vi "Update exp names list.vi"(8 "error in (no error)":errorcluster, 9 "# row":i32, 10 "Experiment in":refnum<class "Experiment.lvclass">, 11 "Control-Client in":refnum<class "Control-Client.lvclass">) -> (0 "error out":errorcluster, 3 "Control-Client out":refnum<class "Control-Client.lvclass">)   [LabVIEW 2019, in "Control-Client.lvclass"]
uses:
  Control-Client.lvclass
  Experiments/Experiment.lvclass
  Control-Client.lvclass/Control-Client.ctl
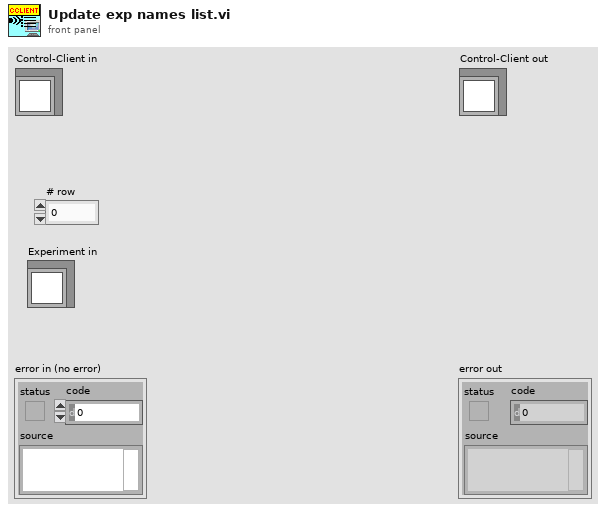
[diagram p1: front panel]
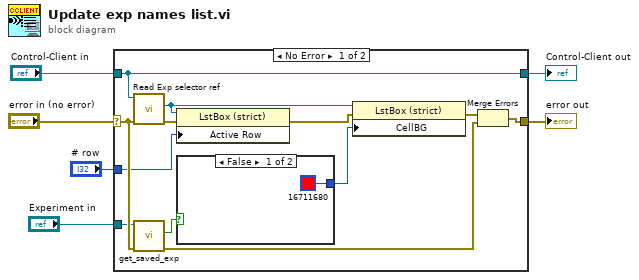
[diagram p0: block diagram]
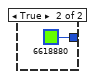
[diagram p2: hidden frame]
diagram:
  n1 = case shown="No Error" "error in (no error)" {
    selector: "error in (no error)" -> [w16 w22]
    tunnel: [w11 w22] -> w5
    tunnel: [w15 w21] -> w3
    tunnel: "Control-Client in" -> [w15 w21]
    tunnel: "Experiment in" -> [w8 _]
    tunnel: "# row" -> [w7 _]
    frame No Error {
      n2 = call "Read Exp selector ref.vi"("error in (no error)"=w16, "Control-Client in"=w15) -> ("error out"=w14:errorcluster, "Exp selector ref"=w18:refnum<vi>)  [unwired: 7 in, 1 out]
      n3 = call "get_saved_exp.vi"("error in (no error)"=w16, "Experiment.lvclass in"=w8) -> ("error out"=w10:errorcluster, "Saved"=w17:bool)  [unwired: 7 in, 1 out]
      n4 = property on="Property Node" class="LstBox (strict)"(reference=w18, error in=w14, "Active Row"=w7) -> (error out=w13:errorcluster)  [unwired: 1 out]
      n5 = case shown="False" w17 {
        tunnel: [u32 16711680 u32 6618880] -> w9
        frame False {
        }
        frame True {
        }
      }
      n6 = property on="Property Node" class="LstBox (strict)"(reference=w18, error in=w13, "CellBG"=w9) -> (error out=w12:errorcluster)  [unwired: 1 out]
      n7 = Merge Errors(w12, w10) -> (w11:errorcluster)
    }
    frame Error {
    }
  }
  "error out" <- w5
  "Control-Client out" <- w3
